vi "Restrict X Range (multiple).vi"(8 "error in (no error)":errorcluster, 9 "X Max":dbl, 10 "X Min":dbl, 11 "XY-data":cluster{"X-array":dbl[], "Y-array":dbl[]}[](array[cluster])) -> (0 "error out":errorcluster, 3 "XY-data out":cluster{"X-array":dbl[], "Y-array":dbl[]}[](array[cluster]) {"Y-array" format="%.2p"; "X-array" format="%.2p"})   [LabVIEW 2016, in "xy_utilities.lvlib"]
doc: "Removes data points that fall outside of the range defined by <b>x min</b> and <b>x max</b>\n\nWire data to the data input to determine the polymorphic instance to use or manually select the instance."
uses:
  xy_utilities.lvlib
  <vilib>/Analysis/6fits.llb/Remove Outliers.vi
  <vilib>/Analysis/6fits.llb/Remove Outliers (Range).vi
  <vilib>/Utility/error.llb/Error Cluster From Error Code.vi
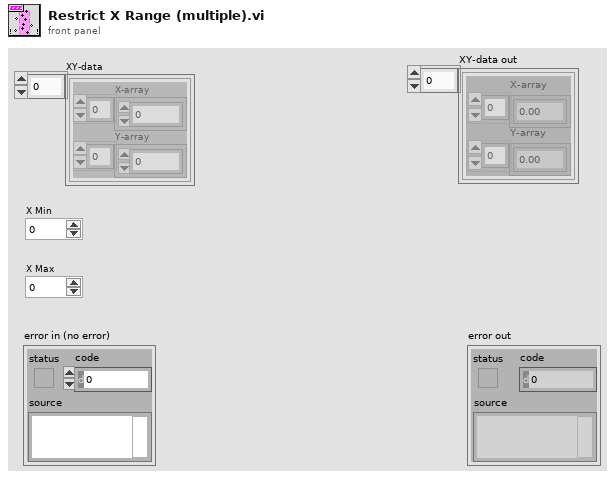
[diagram p1: front panel]
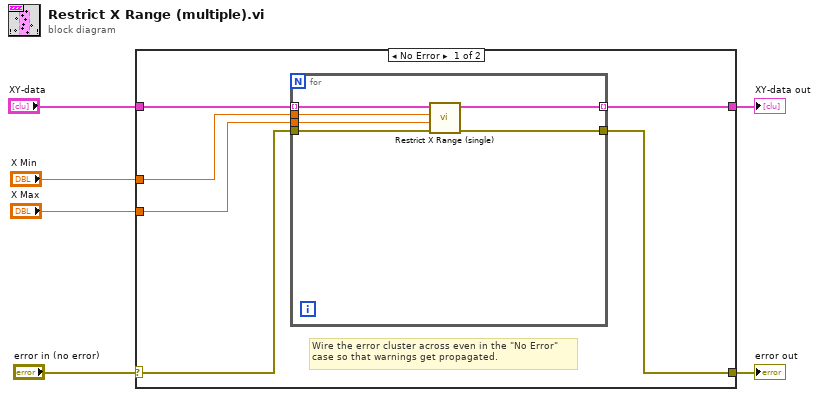
[diagram p0: block diagram]
diagram:
  n1 = case shown="No Error" "error in (no error)" {
    selector: "error in (no error)" -> [w10 w20]
    tunnel: [w9 w20] -> w5
    tunnel: "XY-data" -> [w12 w19]
    tunnel: [w11 w19] -> w3
    tunnel: "X Max" -> [w7 _]
    tunnel: "X Min" -> [w8 _]
    frame No Error {
      # "Wire the error cluster across even in the \"No Error\"\ncase so that warnings get propagated."
      n2 = for {
        tunnel: w12 -> [w18] mode=indexing
        tunnel: [w17] -> w11 mode=indexing
        tunnel: w10 -> [w16]
        tunnel: [w15] -> w9
        tunnel: w8 -> [w14]
        tunnel: w7 -> [w13]
        n3 = call "Restrict X Range (single).vi"("error in (no error)"=w16, "X Max"=w13, "X Min"=w14, "XY-data"=w18) -> ("error out"=w15:errorcluster, "XY-data out"=w17:cluster{"X-array":dbl[], "Y-array":dbl[]})  [unwired: 6 in]
      }
    }
    frame Error {
    }
  }
  "error out" <- w5
  "XY-data out" <- w3
